vi "Timestamp to Excel Serial Date.vi"(11 "Timestamp":timestamp format="%<%x %.3X>T") -> (3 "Excel Serial Date":string)   [LabVIEW 2019, in "Open Xml.lvlib"]
uses:
  Open Xml.lvlib
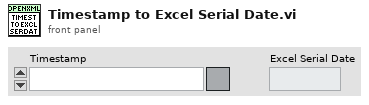
[diagram p1: front panel]
types:
  T1 = typedef "LVDateTimeRec.ctl" = cluster{"fractional second":dbl, "second":i32, "minute":i32, "hour":i32, "day of month":i32, "month":i32, "year":i32, "day of week":i32, "day of year":i32, "DST":i32}
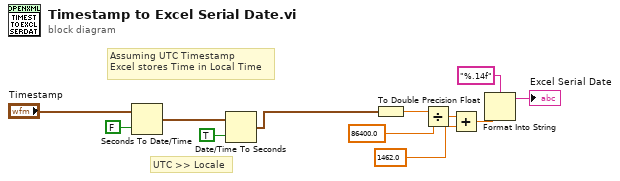
[diagram p0: block diagram]
diagram:
  # "UTC >> Locale"
  # "Assuming UTC Timestamp\nExcel stores Time in Local Time"
  n1 = Seconds To Date/Time(time stamp (now)="Timestamp", to UTC (F)=FALSE) -> (date time rec=w3:T1)
  n2 = Date/Time To Seconds(1:TRUE ("is UTC (F)"), 2:w3) -> (0:w1:timestamp)
  n3 = To Double Precision Float(number=w1) -> (double precision float=w12:dbl)
  n4 = Divide(x=w12, y=86400.0) -> (x/y=w7:dbl)
  n5 = Add(x=w7, y=1462.0) -> (x+y=w10:dbl)
  n6 = Format Into String(format string="%.14f", w10) -> (resulting string=→"Excel Serial Date":string)  [unwired: 2 in, 1 out]
